vi "Get_Method.vi"(6 "Headers":cluster{"Name":string, "Value":string}[](array[cluster]), 8 "error in (no error)":errorcluster, 10 "Endpoint URL":string, 11 "Request in":refnum<class "Request.lvclass">) -> (0 "error out":errorcluster, 2 "Response out":refnum<class "Response.lvclass">, 3 "Request out":refnum<class "Request.lvclass">)   [LabVIEW 2016]
uses:
  Request/Request.lvclass
  Response/Response.lvclass
  Request/PowerShell_Format/Request_Control.ctl
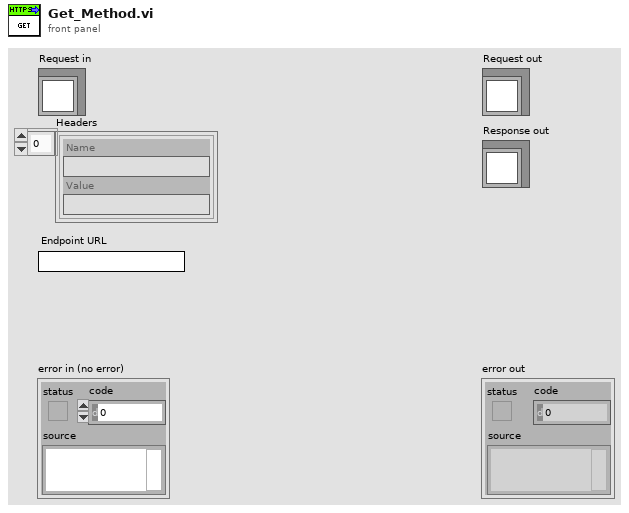
[diagram p1: front panel]
types:
  T1 = typedef "Request.lvclass/Request_Control.ctl" = enum16{"POST", "PATCH_MULTIPART", "POST_MULTIPART", "PATCH", "DELETE", "HEAD", "PUT", "GET"}
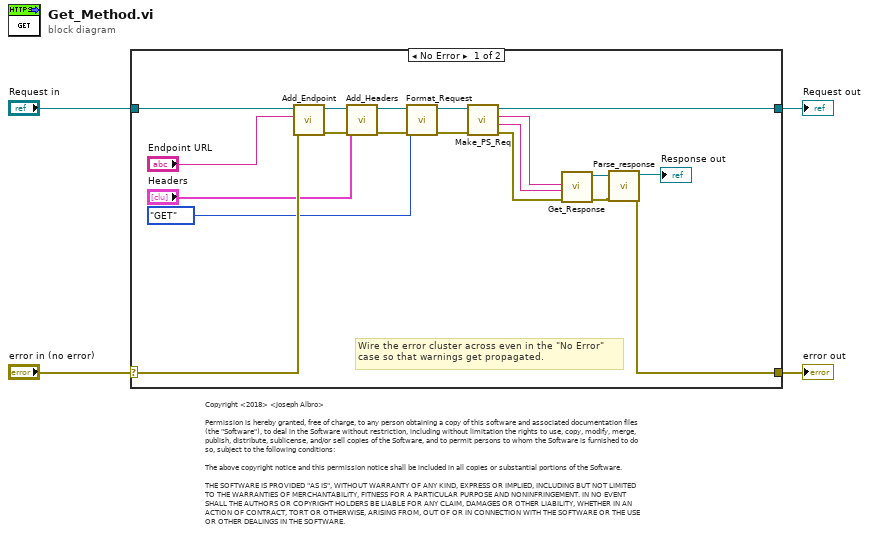
[diagram p0: block diagram]
diagram:
  # "Copyright <2018> <Joseph Albro>\n\nPermission is hereby granted, free of charge, to any person obtaining a copy of this software and associated documentation files (the \"Software\"), to deal in the Software without restriction, including without limitation the rights to use, copy, modify, merge, publish, distribute, sublicense, and/or sell copies of the Software, and to permit persons to whom the Software is furnished to do so, subject to the following conditions:\n\nThe above copyright notice and this permission notice shall be included in all copies or substantial portions of the Software.\n\nTHE SOFTWARE IS PROVIDED \"AS IS\", WITHOUT WARRANTY OF ANY KIND, EXPRESS OR IMPLIED, INCLUDING BUT NOT LIMITED TO THE WARRANTIES OF MERCHANTABILITY, FITNESS FOR A PARTICULAR PURPOSE AND NONINFRINGEMENT. IN NO EVENT SHALL THE AUTHORS OR COPYRIGHT HOLDERS BE LIABLE FOR ANY CLAIM, DAMAGES OR OTHER LIABILITY, WHETHER IN AN ACTION OF CONTRACT, TORT OR OTHERWISE, ARISING FROM, OUT OF OR IN CONNECTION WITH THE SOFTWARE OR THE USE OR OTHER DEALINGS IN THE SOFTWARE."
  n1 = case shown="No Error" "error in (no error)" {
    selector: "error in (no error)" -> [w10 w25]
    tunnel: [w9 w25] -> w3
    tunnel: [w22 w24] -> w1
    tunnel: "Request in" -> [w23 w24]
    frame No Error {
      # "Wire the error cluster across even in the \"No Error\"\ncase so that warnings get propagated."
      n2 = call "Add_Endpoint.vi"("error in (no error)"=w10, "Endpoint URL"="Endpoint URL", "Request in"=w23) -> ("error out"=w18:errorcluster, "Request out"=w19:refnum<class "Request.lvclass">)  [unwired: 7 in]
      n3 = call "Add_Headers.vi"("error in (no error)"=w18, "Headers"="Headers", "Request in"=w19) -> ("error out"=w17:errorcluster, "Request out"=w20:refnum<class "Request.lvclass">)  [unwired: 7 in]
      n4 = call "Format_Request.vi"("error in (no error)"=w17, "Request"=Request_Control."GET", "Request in"=w20) -> ("error out"=w16:errorcluster, "Request out"=w21:refnum<class "Request.lvclass">)  [unwired: 7 in]
      n5 = call "Make_PS_Req.vi"("error in (no error)"=w16, "Request in"=w21) -> ("error out"=w15:errorcluster, "standard error"=w14:string, "standard output"=w13:string, "Request out"=w22:refnum<class "Request.lvclass">)  [unwired: 6 in]
      n6 = call "Get_Response.vi"("error in (no error)"=w15, "PS Error"=w14, "PS Response"=w13) -> ("error out"=w11:errorcluster, "Response out"=w12:refnum<class "Response.lvclass">)  [unwired: 7 in]
      n7 = call "Parse_response.vi"("error in (no error)"=w11, "Response in"=w12) -> ("error out"=w9:errorcluster, "Response out"=→"Response out":refnum<class "Response.lvclass">)  [unwired: 8 in]
    }
    frame Error {
    }
  }
  "error out" <- w3
  "Request out" <- w1
